vi "SafetySystem.vi"() -> ()   [LabVIEW 2018]
uses:
  <vilib>/Platform/TimedLoop/XDataNode/timing_clust.ctl
  <vilib>/Platform/TimedLoop/XDataNode/nitl_modes.ctl
  <vilib>/Platform/TimedLoop/XDataNode/wakeup.ctl
  <vilib>/Modbus/slave/Create Slave Instance (TCP).vi
  <vilib>/Modbus/slave/Modbus Slave.lvclass
  <vilib>/Platform/TimedLoop/XDataNode/XDataNode.xnode
  <vilib>/Platform/TimedLoop/XDataNode/XDNodeRunTimeDep.lvlib
panel:
  in  "stop":bool
  out "TX-SIS-BPCS-ARRAY":bool[](array[boolean])
  out "BPCS-SIM-TX-ARRAY":dbl[](array[numeric])
  out "SIM-SIS-RX-ARRAY":dbl[](array[numeric])
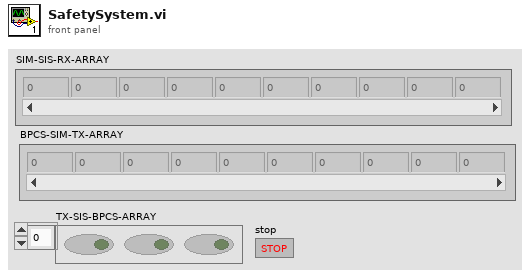
[diagram p1: front panel]
types:
  T1 = typedef "XDNodeRunTimeDep.lvlib/timing_clust.ctl" = cluster{"Expected End [f-1]":u64, "Actual End [f-1]":u64, "Finished Late? [f-1]":bool, "Expected End [i-1]":u64, "Actual End [i-1]":u64, "Finished Late? [i-1]":bool, "Expected Start [i]":u64, "Actual Start [i]":u64, "Expected Start [f]":u64, "Actual Start [f]":u64, "Source Name":string, "Structure Name":string, "Period":i64, "Deadline":i64, "Offset":i64, "Start":i64, "Priority":i32, "Timeout":i32, "Mode":T2, "Wakeup Reason":T3, "Error":errorcluster, "Source Type":string, "Secondary Source Type":string, "Global End Time":u64, "Global Start Time":u64, "Frame Duration":u64, "Iteration Duration":u64, "Assigned CPU":i32, "I/O Scan Engine Mode":u32}
  T2 = typedef "XDNodeRunTimeDep.lvlib/nitl_modes.ctl" = enum32{"No Change", "Process missed periods, maintain original phase", "Discard missed periods, maintain original phase", "Process missed periods, ignore original phase", "Discard missed periods, ignore original phase"}
  T3 = typedef "XDNodeRunTimeDep.lvlib/wakeup.ctl" = enum32{"Normal", "Aborted", "Asynchronous wakeup", "Timing source error", "Timed loop error", "Timeout"}
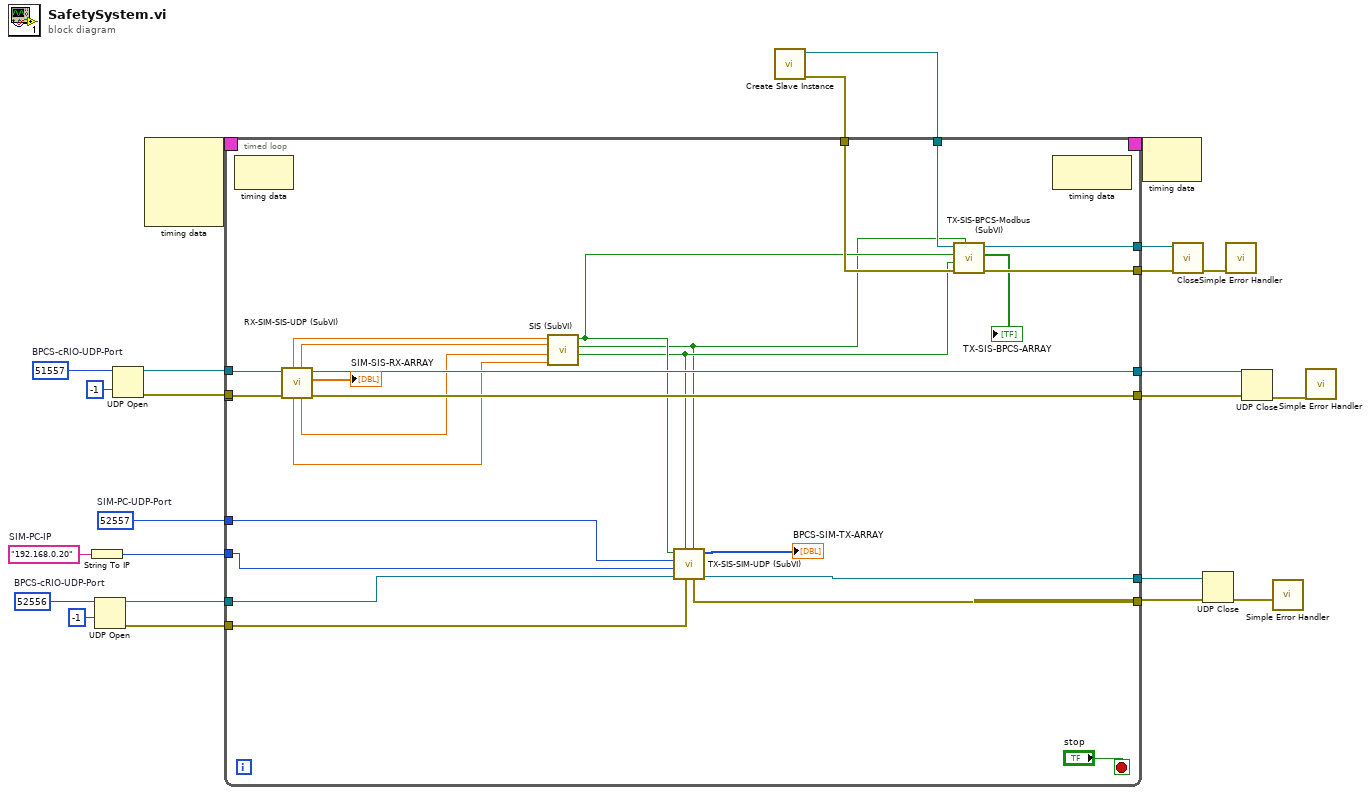
[diagram p0: block diagram]
diagram:
  w14 = u16 52556  # BPCS-cRIO-UDP-Port
  w12 = u16 52557  # SIM-PC-UDP-Port
  w15 = "192.168.0.20"  # SIM-PC-IP
  w21 = u16 51557  # BPCS-cRIO-UDP-Port
  n1 = String To IP(1:w15) -> (0:w11:u32)
  n2 = UDP Open(9:-1 ("timeout ms (25000)"), 11:w14) -> (port=w10:refnum<k16>, 0:w9:errorcluster)  [unwired: 3 in, 1 out]
  n3 = UDP Open(9:-1 ("timeout ms (25000)"), 11:w21) -> (port=w20:refnum<k16>, 0:w19:errorcluster)  [unwired: 3 in, 1 out]
  n4 = node-c288() -> (w24:T1)  [unwired: 4 in]
  n5 = call-poly <vilib>:"Create Slave Instance.vi"() -> ("error out"=w4:errorcluster, "TCP slave instance"=w5:refnum<class "Modbus Slave.lvclass">)  [unwired: 10 in]
  n6 = timed-loop {
    timing: w24 -> [_]
    timing-out: [_] -> w23
    tunnel: w20 -> [w49]
    tunnel: [w48] -> _
    tunnel: w19 -> [w48]
    tunnel: [w47] -> w17
    tunnel: [w46] -> w16
    tunnel: w12 -> [w36]
    tunnel: w11 -> [w35]
    tunnel: w10 -> [w40]
    tunnel: w9 -> [w39]
    tunnel: [w38] -> w6
    tunnel: [w37] -> w7
    tunnel: w5 -> [w33]
    tunnel: w4 -> [w32]
    tunnel: [w28] -> w2
    tunnel: [w27] -> w1
    stop <- "stop" stop-if-true
    n7 = node-c288() -> ()  [unwired: 1 in, 1 out]
    n8 = call "RX-SIM-SIS-UDP (SubVI).vi"("error in (no error)"=w48, "UDP Network Connection in"=w49) -> ("error out"=w46:errorcluster, "SIM-SIS-RX-ARRAY"=→"SIM-SIS-RX-ARRAY":dbl[], "UDP Network Connection out"=w47:refnum<k16>, "SIS-10TI101"=w42:dbl, "SIS-10LI202"=w43:dbl, "SIS-10AI301"=w41:dbl, "SIS-10LI201"=w44:dbl)  [unwired: 3 in]
    n9 = call "SIS (SubVI).vi"("SIS-10AI301"=w41, "SIS-10TI101"=w42, "SIS-10LI202"=w43, "SIS-10LI201"=w44) -> ("SIS-10SDV501"=w30:bool, "SIS-10SDV502"=w29:bool, "SIS-10SDV500"=w31:bool)  [unwired: 5 in]
    n10 = call "TX-SIS-SIM-UDP (SubVI).vi"("SIS-10SDV502"=w29, "error in (no error)"=w39, "SIS-10SDV501"=w30, "UDP Network Connection in"=w40, "SIM-PC-IP"=w35, "SIM-PC-UDP-Port"=w36, "SIS-10SDV500"=w31) -> ("UDP Network Connection out"=w37:refnum<k16>, "BPCS-SIM-TX-ARRAY"=→"BPCS-SIM-TX-ARRAY":i16[], "error out"=w38:errorcluster)  [unwired: 2 in]
    n11 = call "TX-SIS-BPCS-Modbus (SubVI).vi"("SIS-10SDV502"=w29, "error in (no error)"=w32, "SIS-10SDV501"=w30, "SIS-10SDV500"=w31, "Modbus Slave in"=w33) -> ("error out"=w27:errorcluster, "TX-SIS-BPCS-ARRAY"=→"TX-SIS-BPCS-ARRAY":bool[], "Modbus Slave out"=w28:refnum<class "Modbus Slave.lvclass">)  [unwired: 4 in]
    n12 = node-c288() -> ()  [unwired: 1 in, 1 out]
  }
  n13 = node-c288(w23) -> ()  [unwired: 1 out]
  n14 = call-dynamic "Close.vi"("error in (no error)"=w1, "Modbus slave in"=w2) -> ("error out"=w3:errorcluster)  [unwired: 9 in]
  n15 = UDP Close(connection ID=w7, 8:w6) -> (error out=w8:errorcluster)  [unwired: 1 out]
  n16 = call <vilib>:"Simple Error Handler.vi"("error in (no error)"=w3) -> ()  [unwired: 4 in, 5 out]
  n17 = UDP Close(connection ID=w17, 8:w16) -> (error out=w18:errorcluster)  [unwired: 1 out]
  n18 = call <vilib>:"Simple Error Handler.vi"("error in (no error)"=w8) -> ()  [unwired: 4 in, 5 out]
  n19 = call <vilib>:"Simple Error Handler.vi"("error in (no error)"=w18) -> ()  [unwired: 4 in, 5 out]
